vi "SeCrTS-DO waveform to boolean.vi"(11 "DO":waveform(dbl)[](array[waveform])) -> (3 "DO":bool[](array[boolean]))   [LabVIEW 2022 SP3]
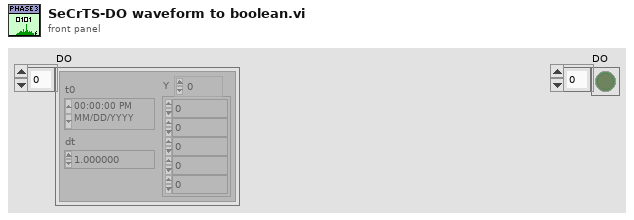
[diagram p1: front panel]
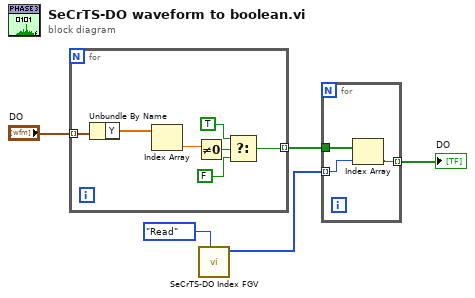
[diagram p0: block diagram]
diagram:
  n1 = for {
    tunnel: "DO" -> [w12] mode=indexing
    tunnel: [w6] -> w5 mode=indexing
    n2 = Unbundle By Name(w12) -> ("Y"=w11:dbl[])
    n3 = Index Array(array=w11) -> (element=w9:dbl)  [unwired: 1 in]
    n4 = Not Equal To 0?(x=w9) -> (x != 0?=w10:bool)
    n5 = Select(t=TRUE, s=w10, f=FALSE) -> (s? t:f=w6:bool)
  }
  n6 = call "SeCrTS-DO Index FGV.vi"("Action"=enum16{"Write", "Read", "Init"}."Read") -> ("Ai Index Element R"=w4:i32[])  [unwired: 10 in]
  n7 = for {
    tunnel: w5 -> [w15]
    tunnel: w4 -> [w14] mode=indexing
    tunnel: [w13] -> w3 mode=indexing
    n8 = Index Array(array=w15, index=w14) -> (element=w13:bool)
  }
  "DO" <- w3
